vi "Check 1-d array.vi"(9 "Array":dbl[][](array[numeric]), 11 "TBL1D":cluster{"X":sgl[], "Y":sgl[]}(xcontrol)) -> (3 "Array 2":dbl[](array[numeric]))   [LabVIEW 2011]
uses:
  XCPCCP TBL1D.xctl
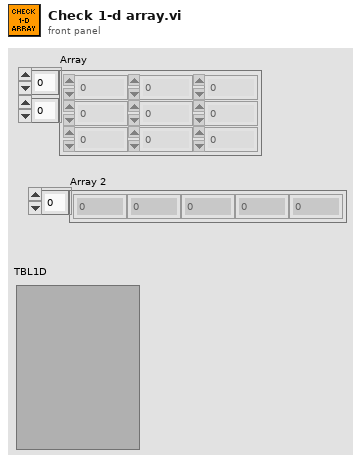
[diagram p1: front panel]
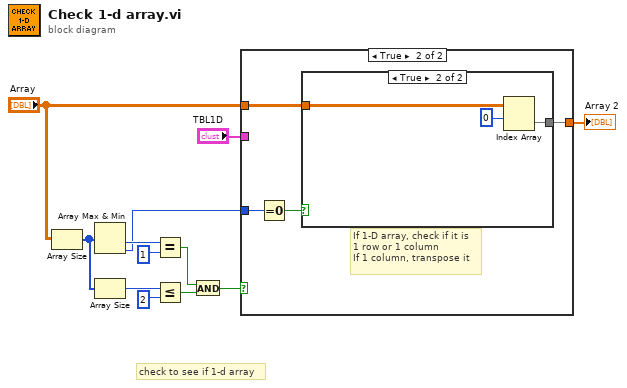
[diagram p0: block diagram]
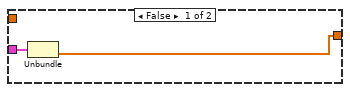
[diagram p2: hidden frame]
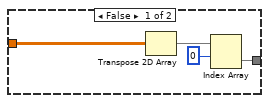
[diagram p3: hidden frame]
diagram:
  # "check to see if 1-d array"
  n1 = Array Size(array="Array") -> (size(s)=w10:i32[])
  n2 = Array Max & Min(array=w10) -> (min value=w11:i32, min index (indices)=w5:i32)  [unwired: 2 out]
  n3 = Array Size(array=w10) -> (size(s)=w9:i32)
  n4 = Equal?(x=w11, y=1) -> (x = y?=w6:bool)
  n5 = Less Or Equal?(x=w9, y=2) -> (x <= y?=w7:bool)
  n6 = And(x=w6, y=w7) -> (x .and. y?=w2:bool)
  n7 = case shown="True" w2 {
    tunnel: w5 -> [_ w18]
    tunnel: "Array" -> [_ w16]
    tunnel: [w14 w15] -> w3
    tunnel: "TBL1D" -> [w13 _]
    frame False {
      n8 = Unbundle(w13) -> ("Y"=w14:sgl[])  [unwired: 1 out]
    }
    frame True {
      # "If 1-D array, check if it is\n1 row or 1 column\nIf 1 column, transpose it"
      n9 = Equal To 0?(x=w18) -> (x = 0?=w17:bool)
      n10 = case shown="True" w17 {
        tunnel: w16 -> [w22 w25]
        tunnel: [w19 w23] -> w15
        frame False {
          n11 = Transpose 2D Array(2D array=w22) -> (transposed array=w21:dbl[][])
          n12 = Index Array(array=w21, index (row)=0) -> (element=w19:dbl[])  [unwired: 1 in]
        }
        frame True {
          n13 = Index Array(array=w25, index (row)=0) -> (element=w23:dbl[])  [unwired: 1 in]
        }
      }
    }
  }
  "Array 2" <- w3
